vi "CVTTraceUpdate.vi"(8 "error in (no error)":errorcluster, 10 "Array":string[](array[string]), 11 "TektronixDPOSimple in":refnum<class "TektronixDPO.lvclass">) -> (0 "error out":errorcluster, 2 "CommandOut":string, 3 "TektronixDPOSimple out":refnum<class "TektronixDPO.lvclass">)   [LabVIEW 2013, in "TektronixDPO.lvclass"]
uses:
  TektronixDPO.lvclass
  TektronixDPO.lvclass/TektronixDPO.ctl
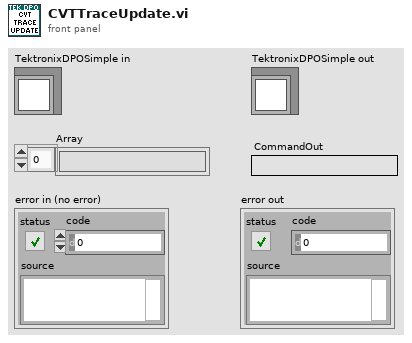
[diagram p1: front panel]
types:
  T1 = cluster{"actualSamples":i32, "absoluteInitialX":dbl, "relativeInitialX":dbl, "xIncrement":dbl, "offset":dbl, "gain":dbl, "reserved1":dbl, "reserved2":dbl}[]
  T2 = typedef "OnOffTypeDef.ctl" = enum16{"off", "on"}
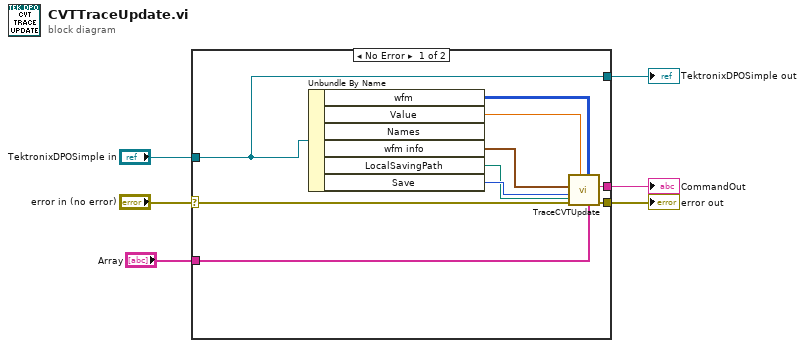
[diagram p0: block diagram]
diagram:
  n1 = case shown="No Error" "error in (no error)" {
    selector: "error in (no error)" -> [w8 w18]
    tunnel: [w11 w18] -> w6
    tunnel: [w10 _] -> w5
    tunnel: "Array" -> [w9 _]
    tunnel: "TektronixDPOSimple in" -> [w7 w17]
    tunnel: [w7 w17] -> w1
    frame No Error {
      n2 = Unbundle By Name ("pressure read")(w7) -> ("wfm"=w16:i16[][], "Value"=w15:dbl, "wfm info"=w14:T1, "LocalSavingPath"=w12:path, "Save"=w13:T2)  [unwired: 1 out]
      n3 = call "TraceCVTUpdate.vi"("Array"=w9, "wfm"=w16, "Settings.LocalSavingPath"=w12, "Number of channels"=w15, "error in (no error)"=w8, "Save"=w13, "wfm info"=w14) -> ("error out"=w11:errorcluster, "String out"=w10:string)  [unwired: 2 in, 1 out]
    }
    frame Error {
    }
  }
  "error out" <- w6
  "CommandOut" <- w5
  "TektronixDPOSimple out" <- w1
